vi "localEngineReference2.vi"   [LabVIEW 2020]
doc: "Use this constant to supply a reference to one of the following items: local PSP Variable Engine, local I/O Variable Engine, local Root PSP Variable Container, or local Root I/O Variable Container."
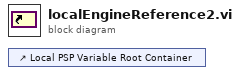
[diagram p0: block diagram]
diagram:
  n1 = control-ref of="Local PSP Variable Root Container"() -> ()  [unwired: 1 out]
